vi "Validate Receive SubAddress.vi"(4 "RT Address (0-30)":u8, 6 "RT 1?":bool, 8 "error in (no error)":errorcluster, 11 "1553 Unit Test in":refnum<class "Remote Terminal.lvclass">) -> (0 "error out":errorcluster, 3 "1553 Unit Test out":refnum<class "Remote Terminal.lvclass">)   [LabVIEW 2020, in "Unit Tests.lvlib" / "Remote Terminal.lvclass"]
uses:
  Remote Terminal.lvclass
  Remote Terminal.lvclass/Remote Terminal.ctl
  <vilib>/addons/_JKI Toolkits/Caraya/classes/Assert/Assert True.vi
  Dependencies/FPGA Interface/FPGA Interface.lvclass
  <vilib>/addons/_JKI Toolkits/Caraya/classes/Assert/Assert.lvclass
  <vilib>/addons/_JKI Toolkits/Caraya/classes/Test/Test.lvclass
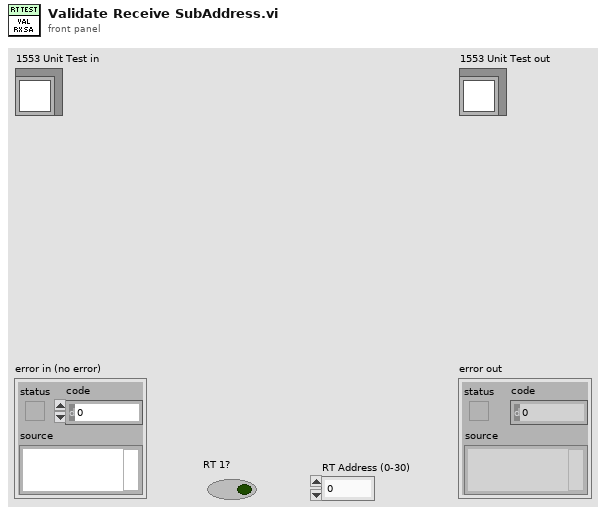
[diagram p1: front panel]
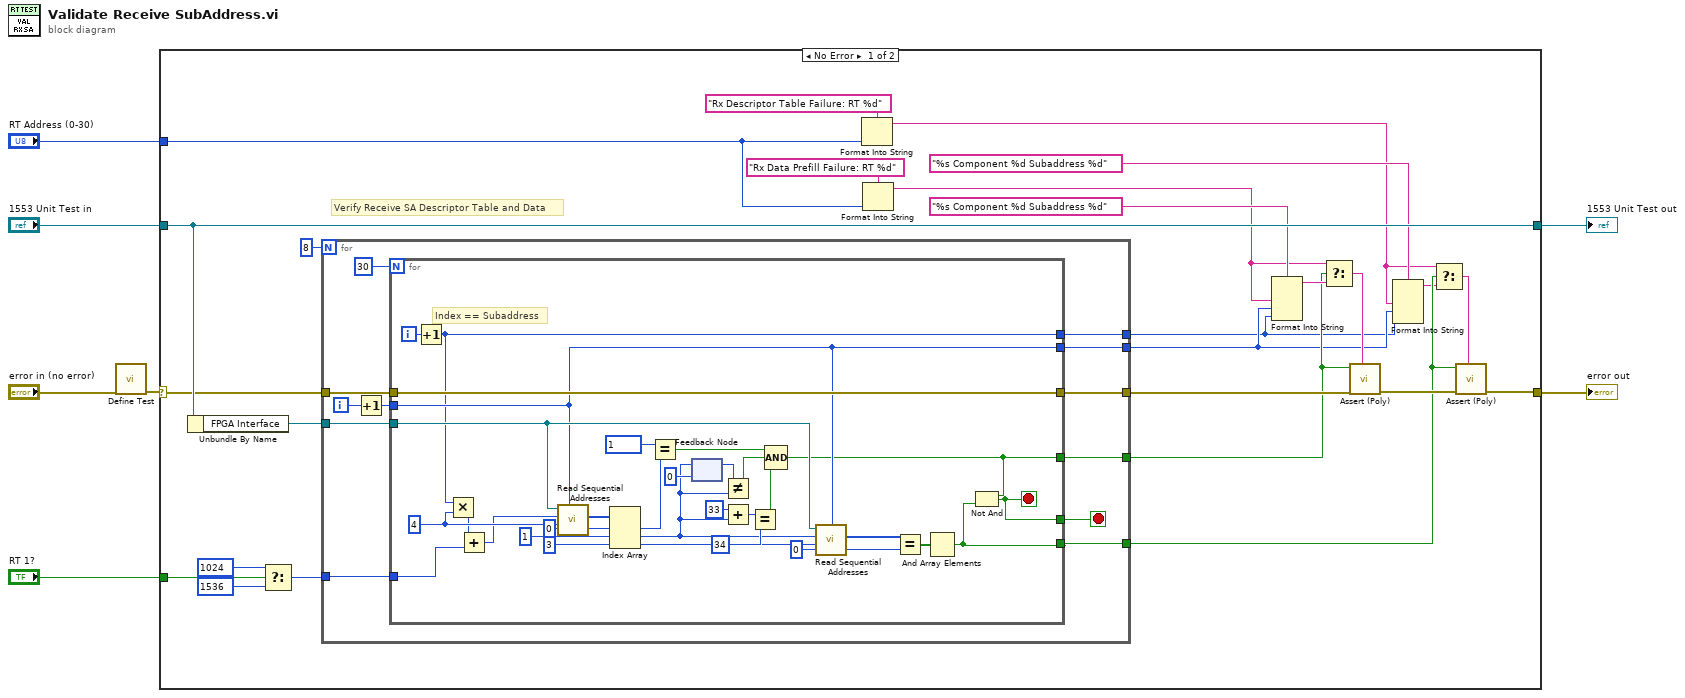
[diagram p0: block diagram]
diagram:
  n1 = call <vilib>:"Define Test.vi"("error in (no error)"="error in (no error)") -> ("error out"=w3:errorcluster)  [unwired: 9 in, 1 out]
  n2 = case shown="No Error" w3 {
    selector: w3 -> [w26 w78]
    tunnel: [w23 w78] -> w7
    tunnel: [w33 w77] -> w5
    tunnel: "1553 Unit Test in" -> [w33 w77]
    tunnel: "RT 1?" -> [w29 _]
    tunnel: "RT Address (0-30)" -> [w12 _]
    frame No Error {
      # "Verify Receive SA Descriptor Table and Data"
      n3 = Unbundle By Name(w33) -> ("FPGA Interface"=w27:refnum<class "FPGA Interface.lvclass">)
      n4 = Select(t=u16 1024, s=w29, f=u16 1536) -> (s? t:f=w28:u16)
      n5 = for {
        N: 8 -> [_]
        tunnel: w28 -> [w34]
        tunnel: w27 -> [w42]
        tunnel: w26 -> [w41]
        tunnel: [w39] -> w24
        tunnel: [w38] -> w9
        tunnel: [w37] -> w8
        tunnel: [w36] -> w20
        tunnel: [w35] -> w17
        i -> [w45]
        stop <- w40 stop-if-true
        n6 = Increment(x=w45) -> (x+1=w43:i32)
        n7 = for {
          N: 30 -> [_]
          tunnel: w43 -> [w73]
          tunnel: w42 -> [w76]
          tunnel: w41 -> [w74]
          tunnel: [w75] -> w35
          tunnel: [w74] -> w39
          tunnel: [w72] -> w36
          tunnel: [w71] -> w40
          tunnel: [w73] -> w38
          tunnel: [w46] -> w37
          tunnel: w34 -> [w48]
          i -> [w51]
          stop <- w71 stop-if-true
          w50 = u16 4 ("x")
          # "Index == Subaddress"
          n8 = Increment(x=w51) -> (x+1=w46:i32)
          n9 = Multiply(x=w46, y=w50) -> (x*y=w49:i32)
          n10 = Add(x=w49, y=w48) -> (x+y=w47:i32)
          n11 = call-dynamic "Read Sequential Addresses.vi"("Target IC (1-8)"=w73, "Addresses to Read"=w50, "Starting Address"=w47, "FPGA Interface in"=w76) -> ("Data"=w52:u16[])  [unwired: 6 in, 1 out]
          n12 = Index Array(array=w52, index #1=0 ("index"), index #2=1 ("index"), index #3=3 ("index")) -> (element #1=w63:u16, element #2=w57:u16, element #3=w59:u16)
          n13 = Equal?(x=u16 1, y=w63) -> (x = y?=w66:bool)
          n14 = feedback #1(u16 0 ("Data")) -> (w65:u16)
          n15 = feedback-in #1(w57) -> ()
          n16 = Not Equal?(x=w65, y=w57) -> (x != y?=w64:bool)
          n17 = Add(x=u16 33, y=w57) -> (x+y=w61:u16)
          n18 = Equal?(x=w61, y=w59) -> (x = y?=w60:bool)
          n19 = Compound Arithmetic op=AND(w66, w64, w60) -> (w72:bool)
          n20 = call-dynamic "Read Sequential Addresses.vi"("Target IC (1-8)"=w73, "Addresses to Read"=u16 34, "Starting Address"=w57, "FPGA Interface in"=w76) -> ("Data"=w53:u16[])  [unwired: 6 in, 1 out]
          n21 = Equal?(x=w53, y=u16 0 ("Data")) -> (x = y?=w54:bool[])
          n22 = And Array Elements(Boolean array=w54) -> (logical AND=w75:bool)
          n23 = Not And(1:w75, 2:w72) -> (0:w71:bool)
        }
      }
      n24 = Format Into String(format string="Rx Descriptor Table Failure: RT %d" ("message (\"\")"), w12) -> (resulting string=w11:string)  [unwired: 2 in, 1 out]
      n25 = Format Into String(format string="Rx Data Prefill Failure: RT %d" ("message (\"\")"), w12) -> (resulting string=w10:string)  [unwired: 2 in, 1 out]
      n26 = Format Into String(format string="%s Component %d Subaddress %d" ("message (\"\")"), w10, w9, w8) -> (resulting string=w21:string)  [unwired: 2 in, 1 out]
      n27 = Select(t=w10, s=w20, f=w21) -> (s? t:f=w19:string)
      n28 = call-poly <vilib>:"Assert (Poly).vi"("Label"=w19, "error in (no error)"=w24, "True?"=w20) -> ("error out"=w25:errorcluster)  [unwired: 7 in, 1 out]
      n29 = Format Into String(format string="%s Component %d Subaddress %d" ("message (\"\")"), w11, w9, w8) -> (resulting string=w16:string)  [unwired: 2 in, 1 out]
      n30 = Select(t=w11, s=w17, f=w16) -> (s? t:f=w15:string)
      n31 = call-poly <vilib>:"Assert (Poly).vi"("Label"=w15, "error in (no error)"=w25, "True?"=w17) -> ("error out"=w23:errorcluster)  [unwired: 7 in, 1 out]
    }
    frame Error {
    }
  }
  "error out" <- w7
  "1553 Unit Test out" <- w5
